vi "ni5660 Sub Set Zoom Settings.vi"(0 "receiver info in":T3, 5 "zoom settings":T2={"zoom FFT settings"={"zoom settings"={"center frequency"=0.0, "zoom"=0, "trim"=1.0}, "FFT settings"={"window"=0, "FFT size"=0}}, "frequency shift"=0.0, "data format"=enum."real"} {"frequency shift" format="%.2f"; "zoom FFT settings"."FFT settings"."window" items=["None ", "Hanning", "Hamming", "Blackman-Harris", "Exact Blackman", "Blackman", "Flat Top", "4 Term B-Harris ", "7 Term B-Harris", "Low Sidelobe"]; "zoom FFT settings"."zoom settings"."trim" min=1.0 format="%.2f"; "zoom FFT settings"."zoom settings"."center frequency" format="%.2f"; "zoom FFT settings"."zoom settings"."zoom" min=1}, 11 "error in (no error)":errorcluster) -> (4 "receiver info out":T3, 15 "error out":errorcluster)   [LabVIEW 2011]
uses:
  <vilib>/addons/Modulation/niScope/controls/mod_Modulation Settings.ctl
  <vilib>/measure/masml.llb/ma_sml_ND Zoom FFT Settings.ctl
  <vilib>/measure/NI_MAPro.lvlib
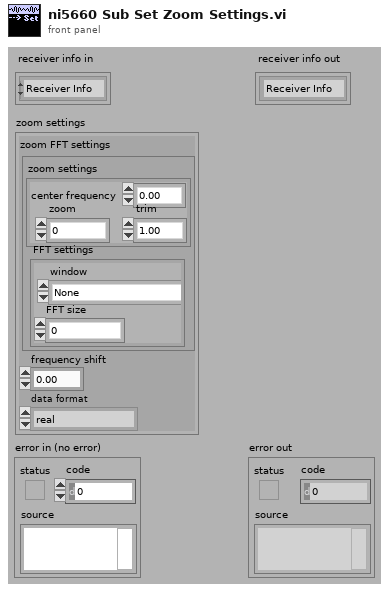
[diagram p1: front panel]
types:
  T1 = typedef "NI_MAPro.lvlib/ma_sml_ND Zoom FFT Settings.ctl" = cluster{"zoom settings":cluster{"center frequency":dbl, "zoom":i32, "trim":dbl}, "FFT settings":cluster{"window":u16, "FFT size":i32}}
  T2 = cluster{"zoom FFT settings":T1, "frequency shift":dbl, "data format":enum16{"real", "complex modulated (array)", "complex modulated (interleaved)"}}
  T3 = typedef "mod_Modulation Settings.ctl" = cluster{enum16{"Receiver Info"}, variant}
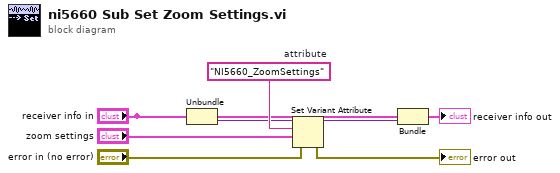
[diagram p0: block diagram]
diagram:
  w8 = "NI5660_ZoomSettings"  # attribute
  n1 = Unbundle("receiver info in") -> (w4:variant)  [unwired: 1 out]
  n2 = Set Variant Attribute(Variant=w4, name=w8, value="zoom settings", error in="error in (no error)") -> (Variant out=w3:variant, error out=→"error out":errorcluster)  [unwired: 1 out]
  n3 = Bundle(cluster="receiver info in", w3) -> (→"receiver info out":T3)  [unwired: 1 in]
